vi "Actor Core.vi"(8 "error in":errorcluster, 11 "Vehicle Position Simulation in":refnum<class "Vehicle Position Simulation.lvclass">) -> (0 "error out":errorcluster, 3 "Actor out":refnum<class "Actor.lvclass">)   [LabVIEW 2019, in "Vehicle Position Simulation.lvlib" / "Vehicle Position Simulation.lvclass"]
doc: "(<B>Filename</B>: Actor Framework.lvlib:Actor.lvclass:Actor Core.vi)\n\nReceives messages to the actor, reacts to them, and initiates any error handling that may shut the actor down.\n\nDescendant classes may override this VI to append parallel tasks for the actor to complete while it handles messages. Overrides use the Call Parent Method node."
uses:
  Vehicle Position Simulation.lvclass
  <vilib>/ActorFramework/Actor/Actor.lvclass
  <vilib>/ActorFramework/Stop Msg/Stop Msg.lvclass
  Abstract Vehicle Position Interface/Abstract Vehicle Position Interface/Vehicle Position Interface.lvclass
  C:/Program Files (x86)/National Instruments/LabVIEW 2019/vi.lib/ActorFramework/Actor/Actor.lvclass
panel:
  out "Vehicle Position Simulation":u32(slide) scale=0.0..4.0
  # "UI1"
  # "UI4."
  # "Entry"
  # "Station1"
  # "Station2"
  # "Station3"
  # "Exit"
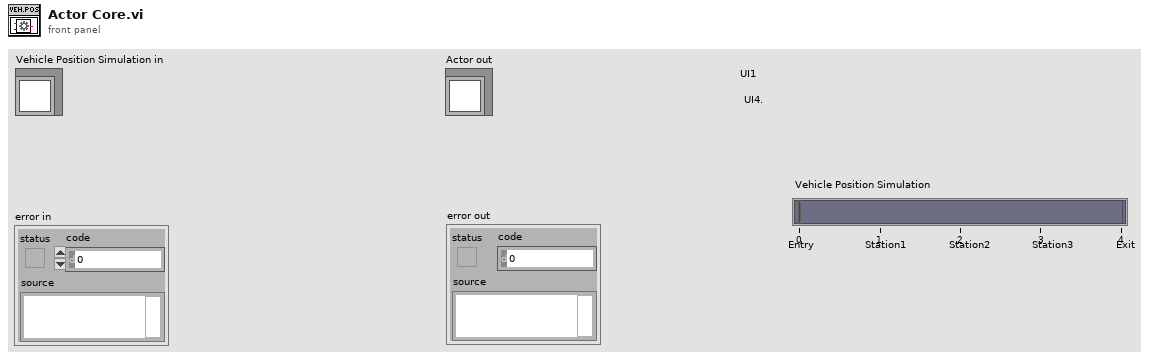
[diagram p1: front panel]
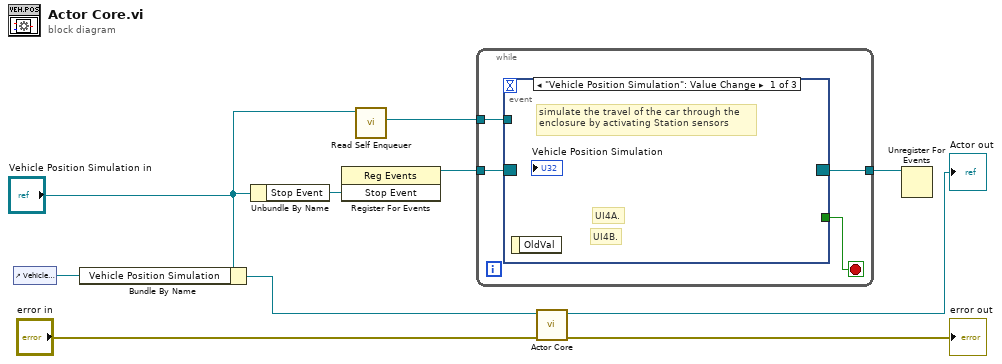
[diagram p0: block diagram]
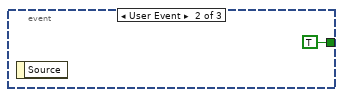
[diagram p2: hidden frame]
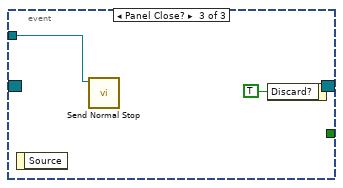
[diagram p3: hidden frame]
diagram:
  n1 = control-ref of="Vehicle Position Simulation"() -> (w6:refnum<vi>)
  n2 = Bundle By Name(cluster="Vehicle Position Simulation in", "Vehicle Position Simulation"=w6) -> (w7:refnum<class "Vehicle Position Simulation.lvclass">)
  n3 = Unbundle By Name("Vehicle Position Simulation in") -> ("Stop Event"=w1:refnum<user-event>)
  n4 = register-events(w1) -> (reference out=w5:refnum<event-registration>)  [unwired: 2 in, 1 out]
  n5 = call <vilib>:"Read Self Enqueuer.vi"("Actor"="Vehicle Position Simulation in") -> ("Self Enqueuer"=w3:refnum<class "Message Enqueuer.lvclass">)  [unwired: 10 in]
  n6 = while {
    tunnel: w5 -> [w13]
    tunnel: [w12] -> w4
    tunnel: w3 -> [w11]
    stop <- w14 stop-if-true
    n7 = event shown="[0] \"Vehicle Position Simulation\": Value Change" {
      selector: w13 -> [_ _ _]
      dyn-events: [_ _ _] -> w12
      timeout: _ -> [_ _ _]
      tunnel: [_ TRUE _] -> w14
      tunnel: w11 -> [_ _ w17]
      event "Vehicle Position Simulation": Value Change {
        # "simulate the travel of the car through the\nenclosure by activating Station sensors"
        # "UI4B."
        # "UI4A."
        n8 = event-data() -> ()  [unwired: 1 in, 1 out]
      }
      event User Event {
        n9 = event-data() -> ()  [unwired: 1 in, 1 out]
      }
      event Panel Close? {
        n10 = event-data() -> ()  [unwired: 1 in, 1 out]
        n11 = call <vilib>:"Send Normal Stop.vi"("Message Enqueuer"=w17) -> ()  [unwired: 10 in, 1 out]
        n12 = event-data("Discard?"=TRUE) -> ()  [unwired: 1 in, 1 out]
      }
    }
  }
  n13 = call-parent "Actor Core.vi"("error in"="error in", "Actor in"=w7) -> ("error out"=→"error out":errorcluster, "Actor out"=→"Actor out":refnum<class "Actor.lvclass">)  [unwired: 8 in]
  n14 = Unregister For Events(event registration refnum=w4) -> ()  [unwired: 1 in, 1 out]
